vi "Test.vi"() -> ()   [LabVIEW 2023]
panel:
  out "data out":string
  out "error out":errorcluster
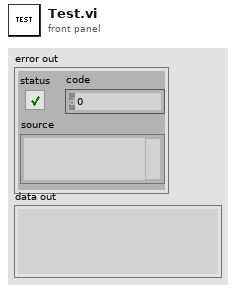
[diagram p1: front panel]
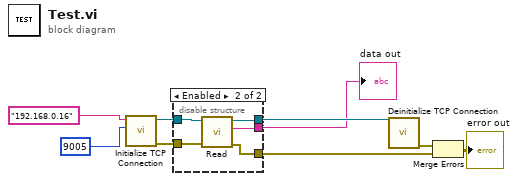
[diagram p0: block diagram]
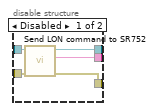
[diagram p2: hidden frame]
diagram:
  n1 = call "Initialize TCP Connection.vi"("Port"=u16 9005, "IP address"="192.168.0.16") -> ("error out"=w6:errorcluster, "TCP Network Connection out"=w7:refnum<k5>)  [unwired: 8 in]
  n2 = disable-structure shown="Enabled" {
    disable-tunnel: w7 -> [w14 w19]
    disable-tunnel: w6 -> [w13 w16]
    disable-tunnel: [w12 w18] -> w5
    disable-tunnel: [w11 w15] -> w3
    disable-tunnel: [w10 w17] -> w1
    frame Disabled {
      n3 = call "Send LON command to SR752.vi"("error in"=w13, "TCP Network Connection in"=w14) -> ("error out"=w11:errorcluster, "data out"=w10:string, "TCP Network Connection out"=w12:refnum<k5>)  [unwired: 7 in]
    }
    frame Enabled {
      n4 = call "Read.vi"("error in"=w16, "TCP in"=w19) -> ("error out"=w15:errorcluster, "ASCII QR Code"=w17:string, "TCP Network Connection out"=w18:refnum<k5>)  [unwired: 7 in]
    }
  }
  "data out" <- w1
  n5 = call "Deinitialize TCP Connection.vi"("TCP Network Connection in"=w5) -> ("error out"=w4:errorcluster)  [unwired: 10 in]
  n6 = Merge Errors(w4, w3) -> (→"error out":errorcluster)
